vi "Castling.vi"(1 "Castling State":bool[][](array[boolean]), 2 "Black/White Turn (T/F)":bool, 3 "Board":i32[][](array[numeric])=[[-3, 0, 0, 0, -1, 0, 0, 0], [-6, -6, -6, -6, -6, -6, -6, -6], [0, 0, 0, 0, 0, 0, 0, 0], [0, 0, 0, 0, 0, 0, 0, 0], [0, 0, 0, 0, 0, 0, 0, 0], [0, 0, 0, 0, 0, 0, 0, 0], [6, 6, 6, 6, 6, 6, 6, 6], [3, 0, 0, 0, 1, 0, 0, 3]], 4 "pieceIndex":i32) -> (0 "Castling position":bool[][](array[boolean]))   [LabVIEW 2014]
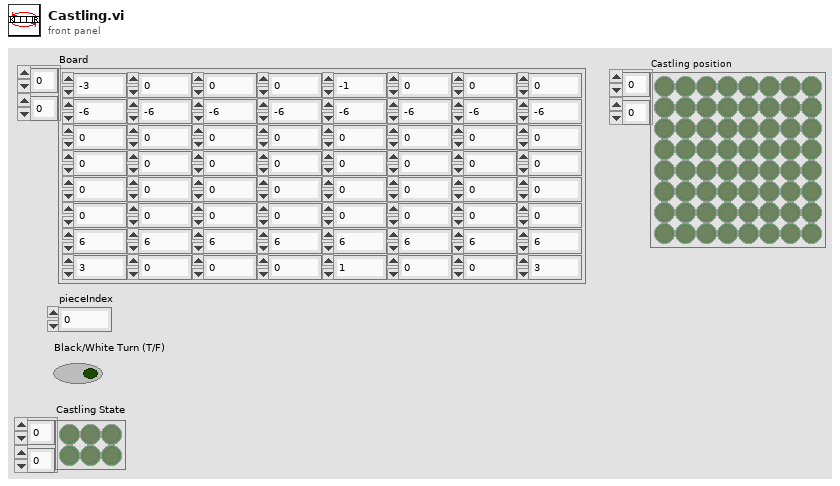
[diagram p1: front panel]
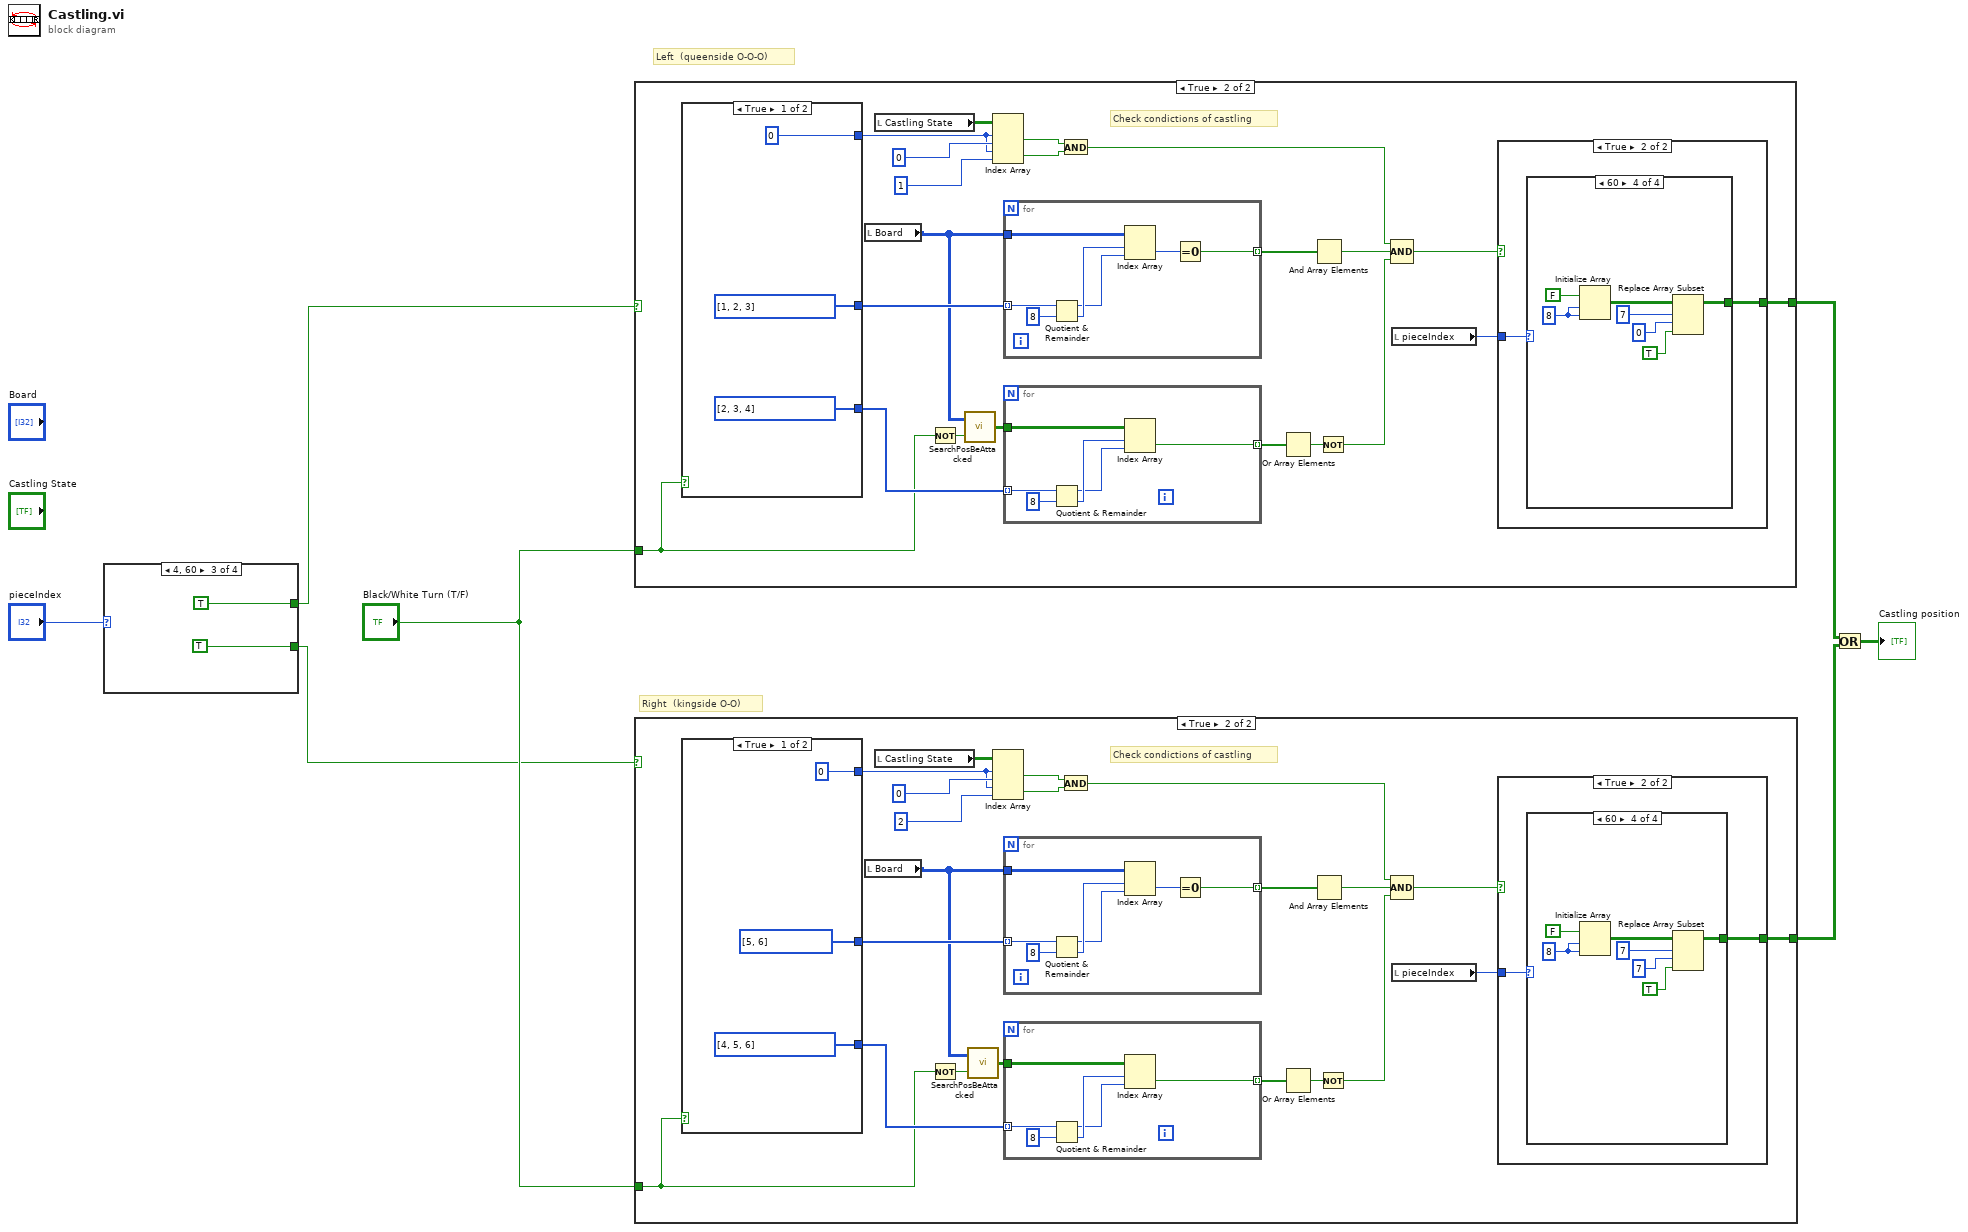
[diagram p0: block diagram]
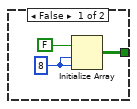
[diagram p2: hidden frame]
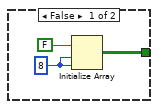
[diagram p3: hidden frame]
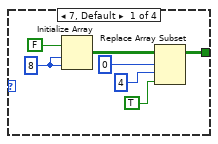
[diagram p4: hidden frame]
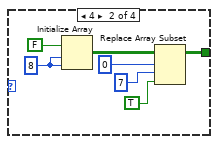
[diagram p5: hidden frame]
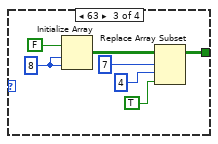
[diagram p6: hidden frame]
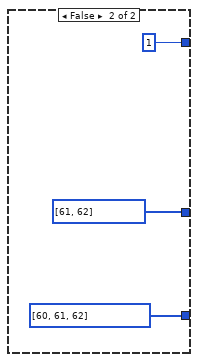
[diagram p7: hidden frame]
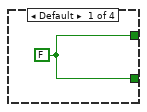
[diagram p8: hidden frame]
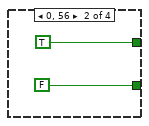
[diagram p9: hidden frame]
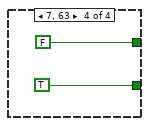
[diagram p10: hidden frame]
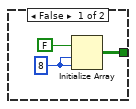
[diagram p11: hidden frame]
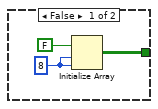
[diagram p12: hidden frame]
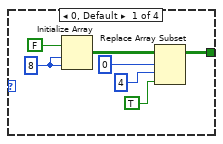
[diagram p13: hidden frame]
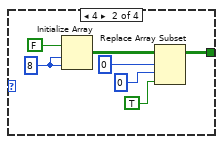
[diagram p14: hidden frame]
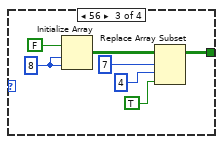
[diagram p15: hidden frame]
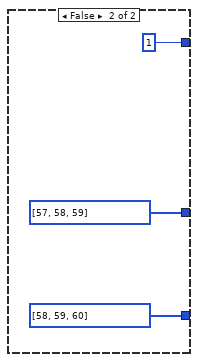
[diagram p16: hidden frame]
diagram:
  # "Right  (kingside O-O)"
  # "Left  (queenside O-O-O)"
  n1 = case shown="4, 60" "pieceIndex" {
    tunnel: [w8 TRUE TRUE FALSE] -> w6
    tunnel: [w8 FALSE TRUE TRUE] -> w1
    frame Default {
      w8 = FALSE
    }
    frame 0, 56 {
    }
    frame 4, 60 {
    }
    frame 7, 63 {
    }
  }
  n2 = case shown="True" w6 {
    tunnel: "Black/White Turn (T/F)" -> [_ w24]
    tunnel: [w15 w18] -> w4
    frame False {
      w16 = 8
      n3 = Initialize Array(FALSE, w16, w16) -> (w15:bool[][])
    }
    frame True {
      # "Check condictions of castling"
      n4 = case shown="True" w24 {
        tunnel: [i32[] [1, 2, 3] i32[] [57, 58, 59]] -> w35
        tunnel: [i32[] [2, 3, 4] i32[] [58, 59, 60]] -> w33
        tunnel: [0 1] -> w25
        frame True {
        }
        frame False {
        }
      }
      n5 = local read "Board"() -> (w32:i32[][])
      n6 = local read "Castling State"() -> (w36:bool[][])
      n7 = Not(x=w24) -> (.not. x?=w30:bool)
      n8 = call "SearchPosBeAttacked.vi"("Black/White (T/F)"=w30, "Board"=w32) -> ("AttackablePosition"=w31:bool[][])
      n9 = Index Array(array=w36, index (row) #1=w25, index (col) #1=0, index (row) #2=w25, index (col) #2=1) -> (element #1=w38:bool, element #2=w37:bool)
      n10 = for {
        tunnel: w35 -> [w83] mode=indexing
        tunnel: w32 -> [w81]
        tunnel: [w78] -> w34 mode=indexing
        n11 = Quotient & Remainder(x=w83, y=8) -> (x-y*floor(x/y)=w80:i32, floor(x/y)=w82:i32)
        n12 = Index Array(array=w81, index (row)=w82, index (col)=w80) -> (element=w79:i32)
        n13 = Equal To 0?(x=w79) -> (x = 0?=w78:bool)
      }
      n14 = for {
        tunnel: w33 -> [w76] mode=indexing
        tunnel: [w72] -> w29 mode=indexing
        tunnel: w31 -> [w73]
        n15 = Quotient & Remainder(x=w76, y=8) -> (x-y*floor(x/y)=w74:i32, floor(x/y)=w75:i32)
        n16 = Index Array(array=w73, index (row)=w75, index (col)=w74) -> (element=w72:bool)
      }
      n17 = And(x=w38, y=w37) -> (x .and. y?=w21:bool)
      n18 = Or Array Elements(Boolean array=w29) -> (logical OR=w28:bool)
      n19 = And Array Elements(Boolean array=w34) -> (logical AND=w22:bool)
      n20 = Not(x=w28) -> (.not. x?=w23:bool)
      n21 = Compound Arithmetic op=AND(w21, w22, w23) -> (w20:bool)
      n22 = local read "pieceIndex"() -> (w19:i32)
      n23 = case shown="True" w20 {
        tunnel: w19 -> [_ w43]
        tunnel: [w39 w42] -> w18
        frame False {
          w40 = 8
          n24 = Initialize Array(FALSE, w40, w40) -> (w39:bool[][])
        }
        frame True {
          n25 = case shown="60" w43 {
            tunnel: [w44 w51 w58 w65] -> w42
            frame 0, Default {
              w49 = 8
              n26 = Initialize Array(FALSE, w49, w49) -> (w48:bool[][])
              n27 = Replace Array Subset(array=w48, new element=TRUE, index (row)=0, index (col)=4 ("disabled index (col)")) -> (w44:bool[][])
            }
            frame 4 {
              w56 = 8
              n28 = Initialize Array(FALSE, w56, w56) -> (w55:bool[][])
              n29 = Replace Array Subset(array=w55, new element=TRUE, index (row)=0, index (col)=0 ("disabled index (col)")) -> (w51:bool[][])
            }
            frame 56 {
              w63 = 8
              n30 = Initialize Array(FALSE, w63, w63) -> (w62:bool[][])
              n31 = Replace Array Subset(array=w62, new element=TRUE, index (row)=7, index (col)=4 ("disabled index (col)")) -> (w58:bool[][])
            }
            frame 60 {
              w70 = 8
              n32 = Initialize Array(FALSE, w70, w70) -> (w69:bool[][])
              n33 = Replace Array Subset(array=w69, new element=TRUE, index (row)=7, index (col)=0 ("disabled index (col)")) -> (w65:bool[][])
            }
          }
        }
      }
    }
  }
  n34 = case shown="True" w1 {
    tunnel: "Black/White Turn (T/F)" -> [_ w100]
    tunnel: [w91 w94] -> w5
    frame False {
      w92 = 8
      n35 = Initialize Array(FALSE, w92, w92) -> (w91:bool[][])
    }
    frame True {
      # "Check condictions of castling"
      n36 = case shown="True" w100 {
        tunnel: [i32[] [5, 6] i32[] [61, 62]] -> w111
        tunnel: [i32[] [4, 5, 6] i32[] [60, 61, 62]] -> w109
        tunnel: [0 1] -> w101
        frame True {
        }
        frame False {
        }
      }
      n37 = local read "Board"() -> (w108:i32[][])
      n38 = local read "Castling State"() -> (w112:bool[][])
      n39 = Not(x=w100) -> (.not. x?=w106:bool)
      n40 = call "SearchPosBeAttacked.vi"("Black/White (T/F)"=w106, "Board"=w108) -> ("AttackablePosition"=w107:bool[][])
      n41 = Index Array(array=w112, index (row) #1=w101, index (col) #1=0, index (row) #2=w101, index (col) #2=2) -> (element #1=w114:bool, element #2=w113:bool)
      n42 = for {
        tunnel: w111 -> [w159] mode=indexing
        tunnel: w108 -> [w157]
        tunnel: [w154] -> w110 mode=indexing
        n43 = Quotient & Remainder(x=w159, y=8) -> (x-y*floor(x/y)=w156:i32, floor(x/y)=w158:i32)
        n44 = Index Array(array=w157, index (row)=w158, index (col)=w156) -> (element=w155:i32)
        n45 = Equal To 0?(x=w155) -> (x = 0?=w154:bool)
      }
      n46 = for {
        tunnel: w109 -> [w152] mode=indexing
        tunnel: [w148] -> w105 mode=indexing
        tunnel: w107 -> [w149]
        n47 = Quotient & Remainder(x=w152, y=8) -> (x-y*floor(x/y)=w150:i32, floor(x/y)=w151:i32)
        n48 = Index Array(array=w149, index (row)=w151, index (col)=w150) -> (element=w148:bool)
      }
      n49 = And(x=w114, y=w113) -> (x .and. y?=w97:bool)
      n50 = Or Array Elements(Boolean array=w105) -> (logical OR=w104:bool)
      n51 = And Array Elements(Boolean array=w110) -> (logical AND=w98:bool)
      n52 = Not(x=w104) -> (.not. x?=w99:bool)
      n53 = Compound Arithmetic op=AND(w97, w98, w99) -> (w96:bool)
      n54 = local read "pieceIndex"() -> (w95:i32)
      n55 = case shown="True" w96 {
        tunnel: w95 -> [_ w119]
        tunnel: [w115 w118] -> w94
        frame False {
          w116 = 8
          n56 = Initialize Array(FALSE, w116, w116) -> (w115:bool[][])
        }
        frame True {
          n57 = case shown="60" w119 {
            tunnel: [w120 w127 w134 w141] -> w118
            frame 7, Default {
              w125 = 8
              n58 = Initialize Array(FALSE, w125, w125) -> (w124:bool[][])
              n59 = Replace Array Subset(array=w124, new element=TRUE, index (row)=0, index (col)=4 ("disabled index (col)")) -> (w120:bool[][])
            }
            frame 4 {
              w132 = 8
              n60 = Initialize Array(FALSE, w132, w132) -> (w131:bool[][])
              n61 = Replace Array Subset(array=w131, new element=TRUE, index (row)=0, index (col)=7 ("disabled index (col)")) -> (w127:bool[][])
            }
            frame 63 {
              w139 = 8
              n62 = Initialize Array(FALSE, w139, w139) -> (w138:bool[][])
              n63 = Replace Array Subset(array=w138, new element=TRUE, index (row)=7, index (col)=4 ("disabled index (col)")) -> (w134:bool[][])
            }
            frame 60 {
              w146 = 8
              n64 = Initialize Array(FALSE, w146, w146) -> (w145:bool[][])
              n65 = Replace Array Subset(array=w145, new element=TRUE, index (row)=7, index (col)=7 ("disabled index (col)")) -> (w141:bool[][])
            }
          }
        }
      }
    }
  }
  n66 = Or(x=w4, y=w5) -> (x .or. y?=→"Castling position":bool[][])
